vi "Primitive equality check.vi"(7 "<Final element name on JSON path>":string, 8 "error in (no error)":errorcluster, 10 "<Upper cluster level>":variant, 11 "<New element to be processed>":variant) -> (0 "error out":errorcluster, 2 "Equal and clusters?":bool, 3 "<Queried object from upper cluster level>":variant)   [LabVIEW 2015]
uses:
  <vilib>/Utility/Data Type/Type Definitions/Data Type.ctl
  <vilib>/Utility/Data Type/NI_Data Type.lvlib
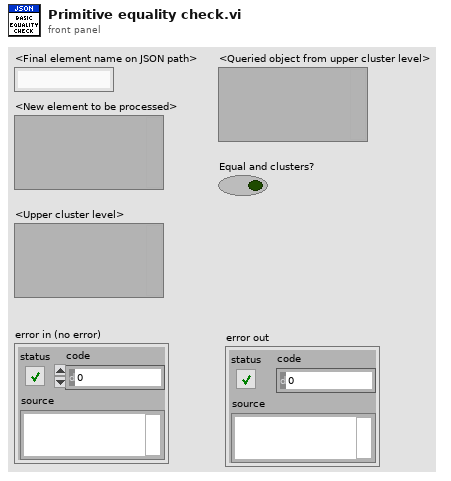
[diagram p1: front panel]
types:
  T1 = typedef "NI_Data Type.lvlib/Data Type.ctl" = enum8{"Invalid Type", "Void", "I8", "I16", "I32", "I64", "U8", "U16", "U32", "U64", "Single Float", "Double Float", "Extended Float", "Single Complex", "Double Complex", "Extended Complex", "Enum U8", "Enum U16", "Enum U32", "Enum U64", "Single Float With Unit", "Double Float With Unit", "Extended Float With Unit", "Single Complex with Unit", "Double Complex with Unit", "Extended Complex with Unit", "Boolean", "String", "Path", "Picture", "Tag", "Array", "Cluster", "Variant", "LV Variant", "Waveform", "Timestamp", "Digital Waveform", "Digital Data", "ExpressData", "Refnum", "External Data", "VI", "Poly VI", "LabVIEW Class Instance", "Fixed Point"}
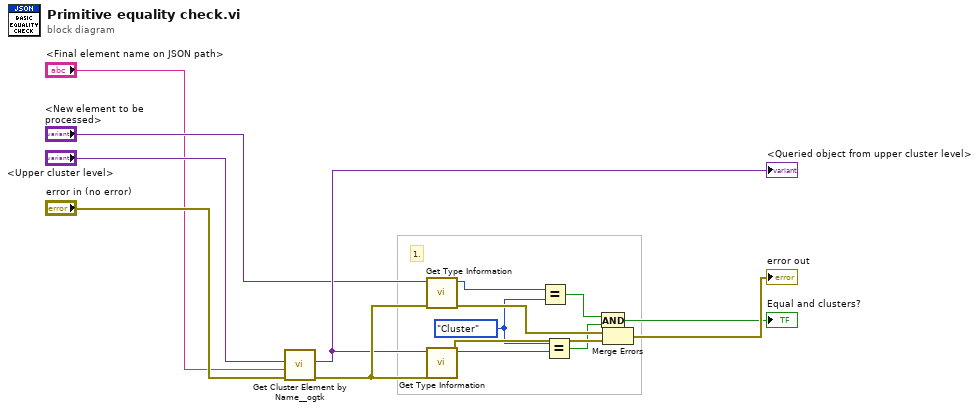
[diagram p0: block diagram]
diagram:
  w12 = Data_Type."Cluster" ("y")
  # "1."
  n1 = call <userlib>:"Get Cluster Element by Name__ogtk.vi"("error in (no error)"="error in (no error)", "Element Name"="<Final element name on JSON path>", "Cluster"="<Upper cluster level>") -> ("error out"=w9:errorcluster, "VElement"=w8:variant)  [unwired: 6 in, 1 out]
  "<Queried object from upper cluster level>" <- w8
  n2 = call <vilib>:"Get Type Information.vi"("error in (no error)"=w9, "Variant"="<New element to be processed>") -> ("error out"=w15:errorcluster, "Type"=w11:T1)  [unwired: 5 in, 3 out]
  n3 = call <vilib>:"Get Type Information.vi"("error in (no error)"=w9, "Variant"=w8) -> ("error out"=w13:errorcluster, "Type"=w10:T1)  [unwired: 5 in, 3 out]
  n4 = Equal?(x=w11, y=w12) -> (x = y?=w3:bool)
  n5 = Equal?(x=w12, y=w10) -> (x = y?=w1:bool)
  n6 = And(x=w3, y=w1) -> (x .and. y?=→"Equal and clusters?":bool)
  n7 = Merge Errors(w15, w13) -> (→"error out":errorcluster)
